vi "LTVUnicycleCtrl_Execute_TrajState.vi"(5 "LTV_Unicycle_Ctrl_Model":T2={"Max linear ctrl effort M/S"=1.0, "Max angular ctrl effort Rad/S"=2.0, "Max Heading Meas Tol Rad"=0.2, "Max X Pos Meas Tol M"=0.0625, "Max Y Pos Meas Tol M"=0.125, "Max Linear Vel M/S"=9.0} {"Max Linear Vel M/S" format="%#_13g"; "Max Y Pos Meas Tol M" format="%#_13g"; "Max X Pos Meas Tol M" format="%#_13g"; "Max Heading Meas Tol Rad" format="%#_13g"; "Max angular ctrl effort Rad/S" format="%#_13g"; "Max linear ctrl effort M/S" format="%#_13g"}, 7 "LTV_Unicycle_Ctrl_Tolerance":T1={"Max Heading Tolerance Rad"=0.2, "Max X Tolerance M"=0.0625, "Max Y Tolerance M"=0.125} {"Max Y Tolerance M" format="%#_13g"; "Max X Tolerance M" format="%#_13g"; "Max Heading Tolerance Rad" format="%#_13g"}, 8 "dT Sec":dbl=0.02, 9 "Enabled":bool=TRUE, 10 "CurrentPose":T4={"TRANSLATION"={"X"=0.0, "Y"=0.0}, "ROTATION"={"VALUE"=0.0, "COS"=1.0, "SIN"=0.0}} {"ROTATION"."SIN" format="%13.4f"; "ROTATION"."COS" format="%13.4f"; "ROTATION"."VALUE" format="%13.4f"; "TRANSLATION"."Y" format="%14.3f"; "TRANSLATION"."X" format="%14.3f"}, 11 "TRAJ_STATE":T3={"TimeSeconds"=0.0, "Velocity"=0.0, "Acceleration"=0.0, "POSE"={"TRANSLATION"={"X"=0.0, "Y"=0.0}, "ROTATION"={"VALUE"=0.0, "COS"=1.0, "SIN"=0.0}}, "Curvature"=0.0} {"POSE"."ROTATION"."SIN" format="%13.4f"; "POSE"."ROTATION"."COS" format="%13.4f"; "POSE"."ROTATION"."VALUE" format="%13.4f"; "POSE"."TRANSLATION"."Y" format="%14.3f"; "POSE"."TRANSLATION"."X" format="%14.3f"}) -> (0 "Error":bool, 1 "out LTV_UNICYCLE_CONTROLLER":T8={"States"=0, "Inputs"=0, "PoseError"={"TRANSLATION"={"X"=0.0, "Y"=0.0}, "ROTATION"={"VALUE"=0.0, "COS"=1.0, "SIN"=0.0}}, "PoseTolerance"={"TRANSLATION"={"X"=0.0, "Y"=0.0}, "ROTATION"={"VALUE"=0.0, "COS"=1.0, "SIN"=0.0}}, "Dt"=0.02, "Enabled"=FALSE, "LQR_K_Table"={"Table Xs"=[], "Table Ys"=[], "MinX"=0.0, "MaxX"=0.0, "ItemCount"=0, "Rows"=0, "Columns"=0}} {"PoseTolerance"."ROTATION"."SIN" format="%13.4f"; "PoseTolerance"."ROTATION"."COS" format="%13.4f"; "PoseTolerance"."ROTATION"."VALUE" format="%13.4f"; "PoseTolerance"."TRANSLATION"."Y" format="%14.3f"; "PoseTolerance"."TRANSLATION"."X" format="%14.3f"; "PoseError"."ROTATION"."SIN" format="%13.4f"; "PoseError"."ROTATION"."COS" format="%13.4f"; "PoseError"."ROTATION"."VALUE" format="%13.4f"; "PoseError"."TRANSLATION"."Y" format="%14.3f"; "PoseError"."TRANSLATION"."X" format="%14.3f"}, 2 "At Reference":bool, 3 "ChassisSpeeds":T7 {"vOmega" format="%10.3f"; "vY" format="%10.3f"; "vX" format="%10.3f"})   [LabVIEW 2019, in "Trajectory_Library.lvlib"]
doc: "The linear time-varying unicycle controller has a similar form to the LQR, but the model used to compute the controller gain is the nonlinear model linearized around the drivetrain's current state.\n\nThis LabVIEW single call function creates and executes the LTV Unicycle controller. \n\n\nInputs:\n - LTVUnicycleCtrl Model -- cluster -- Packed data used to construct the LTV Unicycle control system.\n - LTVUnicycleCtrl Tol -- cluster -- Packed data used to define the tolerance LTV Unicycle control system.\n - Traj State -- Traj State -- The desired trajectory state. contains desired position and speeds (Meters, Radians)\n - Current Pose -- Pose2d -- The current pose. (Meters, Radians)\n - Enabled -- boolean -- If TRUE use closed loop control to calculate desired chassis speeds. If FALSE, outputs the reference speeds directly.\n - dt Sec -- double -- Update time (default: 0.02)\n\nOutputs:\n - Chassis Speed -- chassis speed -- Chassis Speed Demand\n - At Reference -- boolean -- If TRUE, the current position is within the tolerance.\n - Error -- boolean -- If TRUE, an error occured.\n - out LTV UnicycleCtrl -- cluster -- Internal data structure."
uses:
  Trajectory_Library.lvlib
  TypeDef/LTV_UNICYCLE_CONTROLLER.ctl
  TypeDef/POSE2D.ctl
  TypeDef/TRANSLATION2D.ctl
  TypeDef/ROTATION2D.ctl
  TypeDef/FUNCTION_GENERATOR_MATRIX.ctl
  TypeDef/CHASSIS_SPEEDS.ctl
  TypeDef/TRAJ_STATE.ctl
  TypeDef/LTV_UNICYCLE_CONTROLLER_MODEL_PARAMS.CTL
  TypeDef/LTV_UNICYCLE_CONTROLLER_TOLERANCE.CTL
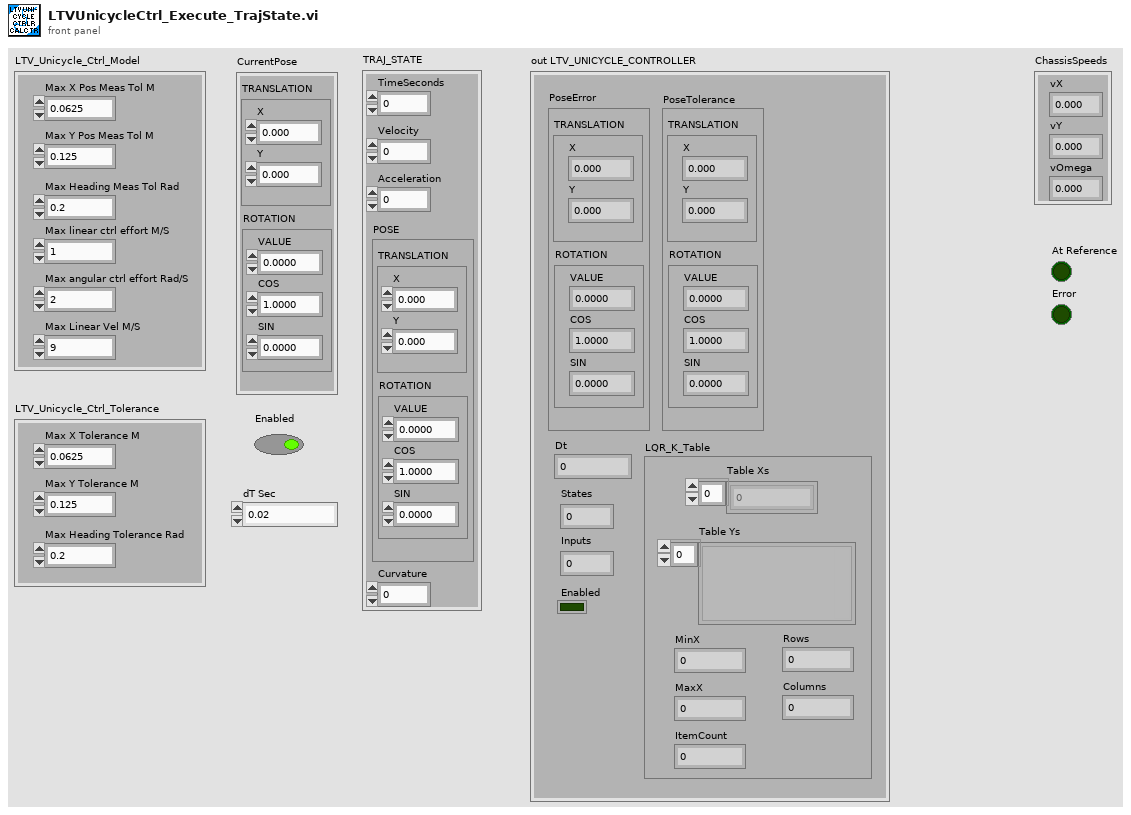
[diagram p1: front panel]
types:
  T1 = typedef "Trajectory_Library.lvlib/LTV_UNICYCLE_CONTROLLER_TOLERANCE.CTL" = cluster{"Max Heading Tolerance Rad":dbl, "Max X Tolerance M":dbl, "Max Y Tolerance M":dbl}
  T2 = typedef "Trajectory_Library.lvlib/LTV_UNICYCLE_CONTROLLER_MODEL_PARAMS.CTL" = cluster{"Max linear ctrl effort M/S":dbl, "Max angular ctrl effort Rad/S":dbl, "Max Heading Meas Tol Rad":dbl, "Max X Pos Meas Tol M":dbl, "Max Y Pos Meas Tol M":dbl, "Max Linear Vel M/S":dbl}
  T3 = typedef "Trajectory_Library.lvlib/TRAJ_STATE.ctl" = cluster{"TimeSeconds":dbl, "Velocity":dbl, "Acceleration":dbl, "POSE":T4, "Curvature":dbl}
  T4 = typedef "Trajectory_Library.lvlib/POSE2D.ctl" = cluster{"TRANSLATION":T5, "ROTATION":T6}
  T5 = typedef "Trajectory_Library.lvlib/TRANSLATION2D.ctl" = cluster{"X":dbl, "Y":dbl}
  T6 = typedef "Trajectory_Library.lvlib/ROTATION2D.ctl" = cluster{"VALUE":dbl, "COS":dbl, "SIN":dbl}
  T7 = typedef "Trajectory_Library.lvlib/CHASSIS_SPEEDS.ctl" = cluster{"vX":dbl, "vY":dbl, "vOmega":dbl}
  T8 = typedef "Trajectory_Library.lvlib/LTV_UNICYCLE_CONTROLLER.ctl" = cluster{"States":i32, "Inputs":i32, "PoseError":T4, "PoseTolerance":T4, "Dt":dbl, "Enabled":bool, "LQR_K_Table":T9}
  T9 = typedef "Trajectory_Library.lvlib/FUNCTION_GENERATOR_MATRIX.ctl" = cluster{"Table Xs":dbl[], "Table Ys":variant[], "MinX":dbl, "MaxX":dbl, "ItemCount":i32, "Rows":i32, "Columns":i32}
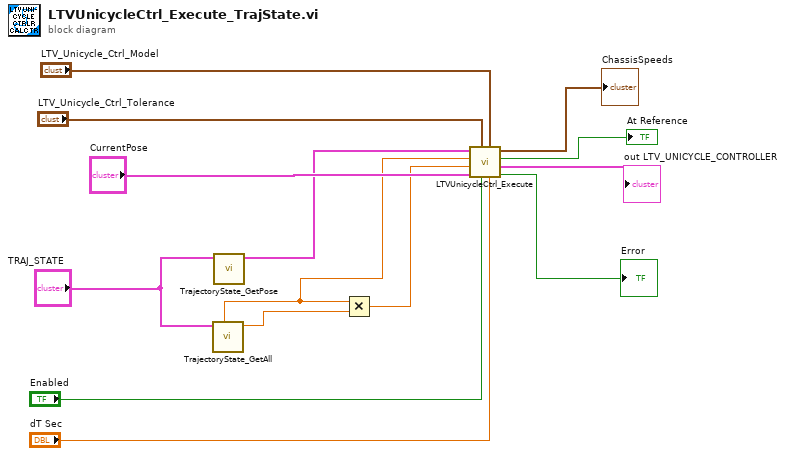
[diagram p0: block diagram]
diagram:
  n1 = call "TrajectoryState_GetAll.vi"("TRAJ_STATE"="TRAJ_STATE") -> ("Curvature"=w8:dbl, "Velocity"=w6:dbl)  [unwired: 4 in, 5 out]
  n2 = call "TrajectoryState_GetPose.vi"("TRAJ_STATE"="TRAJ_STATE") -> ("TrajStatePose"=w10:T4)  [unwired: 10 in]
  n3 = Multiply(x=w6, y=w8) -> (x*y=w5:dbl)
  n4 = call "LTVUnicycleCtrl_Execute.vi"("dT Sec"="dT Sec", "LTV_Unicycle_Ctrl_Model"="LTV_Unicycle_Ctrl_Model", "Enabled"="Enabled", "LTV_Unicycle_Ctrl_Tolerance"="LTV_Unicycle_Ctrl_Tolerance", "CurrentPose"="CurrentPose", "RefAngularVelocity"=w5, "RefLinearVelocity"=w6, "RefPose"=w10) -> ("Error"=→"Error":bool, "out LTV_UNICYCLE_CONTROLLER"=→"out LTV_UNICYCLE_CONTROLLER":T8, "At Reference"=→"At Reference":bool, "ChassisSpeeds"=→"ChassisSpeeds":T7)
